vi "PixyCam_TargetStore.vi"(4 "Operation":enum16{"set", "get"}(ring), 5 "ColorCodeTargets Set":T1[](array[typedef])=[{"Target Type"=0, "Checksum"=0, "Signature Number"=0, "X Center"=0, "Y Center"=0, "Width"=0, "Height"=0, "Angle"=0}] {"Angle" format="%x"; "Height" format="%x"; "Width" format="%x"; "Y Center" format="%x"; "X Center" format="%x"; "Signature Number" format="%x"; "Checksum" format="%x"; "Target Type" items=["PIXY_START_WORD"=43605, "PIXY_START_WORD_CC"=43606, "PIXY_START_WORDX"=21930]}, 6 "StandardTargets Set":T1[](array[typedef])=[{"Target Type"=0, "Checksum"=0, "Signature Number"=0, "X Center"=0, "Y Center"=0, "Width"=0, "Height"=0, "Angle"=0}] {"Angle" format="%x"; "Height" format="%x"; "Width" format="%x"; "Y Center" format="%x"; "X Center" format="%x"; "Signature Number" format="%x"; "Checksum" format="%x"; "Target Type" items=["PIXY_START_WORD"=43605, "PIXY_START_WORD_CC"=43606, "PIXY_START_WORDX"=21930]}, 7 "PixyCamDevRef":T2) -> (1 "ColorCodeTargets Out":T1[](array[typedef]) {"Angle" format="%x"; "Height" format="%x"; "Width" format="%x"; "Y Center" format="%x"; "X Center" format="%x"; "Signature Number" format="%x"; "Checksum" format="%x"; "Target Type" items=["PIXY_START_WORD"=43605, "PIXY_START_WORD_CC"=43606, "PIXY_START_WORDX"=21930]}, 2 "StandardTargets Out":T1[](array[typedef]) {"Angle" format="%x"; "Height" format="%x"; "Width" format="%x"; "Y Center" format="%x"; "X Center" format="%x"; "Signature Number" format="%x"; "Checksum" format="%x"; "Target Type" items=["PIXY_START_WORD"=43605, "PIXY_START_WORD_CC"=43606, "PIXY_START_WORDX"=21930]}, 3 "PixyCamDevRef Out":T2)   [LabVIEW 2016, in "PixyCam_LabVIEW.lvlib"]
uses:
  PixyCam_LabVIEW.lvlib
  PixyCam_DevRef.ctl
  PixyCam_SPI_DevRef.ctl
  <vilib>/Rock Robotics/WPI/SPI/WPI_SPIDevRef.ctl
  <vilib>/Rock Robotics/SystemInterfaces/spilib/spi_bus.ctl
  PixyCam_CommMode.ctl
  PixyCam_TargetData.ctl
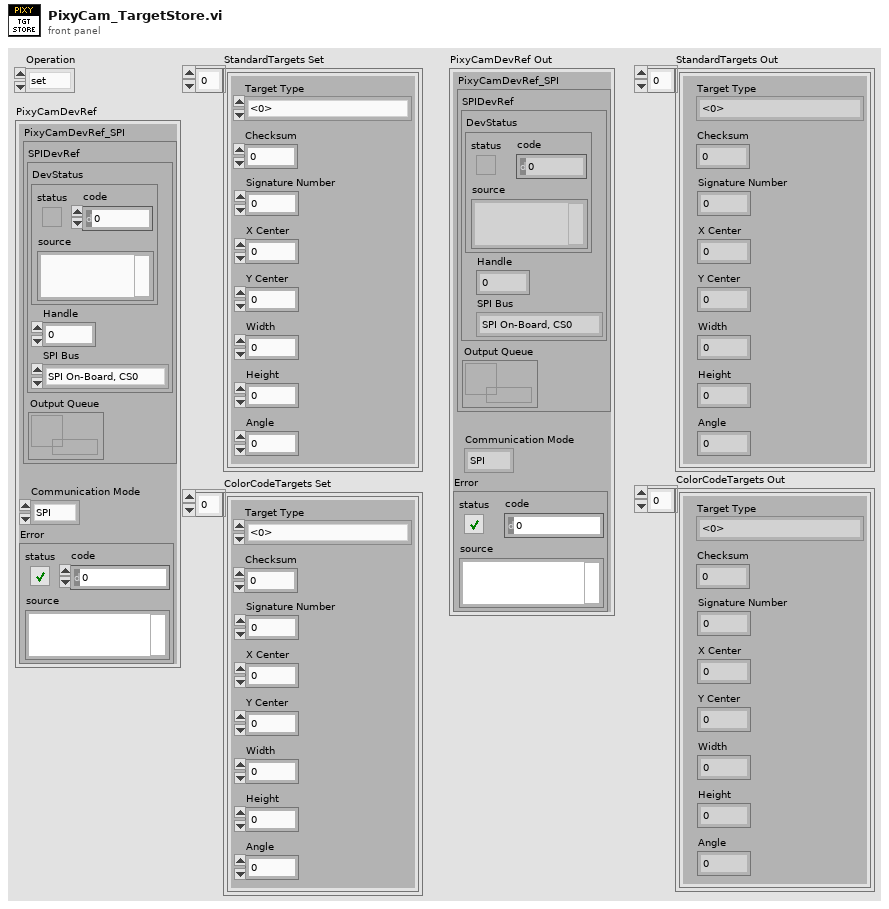
[diagram p1: front panel]
types:
  T1 = typedef "PixyCam_LabVIEW.lvlib/PixyCam_TargetData.ctl" = cluster{"Target Type":u16, "Checksum":u16, "Signature Number":u16, "X Center":u16, "Y Center":u16, "Width":u16, "Height":u16, "Angle":u16}
  T2 = typedef "PixyCam_LabVIEW.lvlib/PixyCam_DevRef.ctl" = cluster{"PixyCamDevRef_SPI":T3, "Communication Mode":T6, "Error":errorcluster}
  T3 = typedef "PixyCam_LabVIEW.lvlib/PixyCam_SPI_DevRef.ctl" = cluster{"SPIDevRef":T4, "Output Queue":refnum<queue>}
  T4 = typedef "WPI_SPIDevRef.ctl" = cluster{"DevStatus":errorcluster, "Handle":i32, "SPI Bus":T5}
  T5 = typedef "spi_bus.ctl" = enum16{"SPI On-Board, CS0", "SPI On-Board, CS1", "SPI On-Board, CS2", "SPI On-Board, CS3", "SPI MXP", "Invalid"}
  T6 = typedef "PixyCam_LabVIEW.lvlib/PixyCam_CommMode.ctl" = enum16{"SPI", "I2C", "UART", "Analog", "Digital"}
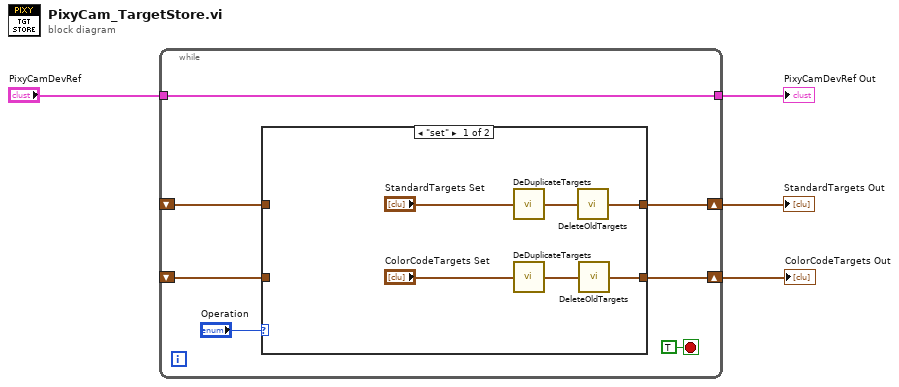
[diagram p0: block diagram]
diagram:
  n1 = while {
    shift-right: [w9] -> w2
    shift-left: _ -> [w5]
    tunnel: "PixyCamDevRef" -> [w8]
    tunnel: [w8] -> w3
    shift-right: [w7] -> w1
    shift-left: _ -> [w6]
    stop <- TRUE stop-if-true
    n2 = case shown="\"set\"" "Operation" {
      tunnel: [w13 w18] -> w9
      tunnel: [w12 w19] -> w7
      tunnel: w6 -> [_ w19]
      tunnel: w5 -> [_ w18]
      frame "set" {
        n3 = call "DeDuplicateTargets.vi"("TargetsIn"="StandardTargets Set") -> ("TargetsOut"=w16:T1[])
        n4 = call "DeDuplicateTargets.vi"("TargetsIn"="ColorCodeTargets Set") -> ("TargetsOut"=w14:T1[])
        n5 = call "DeleteOldTargets.vi"("TargetsIn"=w16) -> ("TargetsOut"=w13:T1[])
        n6 = call "DeleteOldTargets.vi"("TargetsIn"=w14) -> ("TargetsOut"=w12:T1[])
      }
      frame "get", Default {
      }
    }
  }
  "PixyCamDevRef Out" <- w3
  "StandardTargets Out" <- w2
  "ColorCodeTargets Out" <- w1
